vi "Mark as Source Only.vi"() -> ()   [LabVIEW 2011]
uses:
  <vilib>/regexp/Match Regular Expression.xnode
panel:
  in  "Interactive?":bool
  out "errors":path[](array[path])
  out "stripped":path[](array[path])
  out "Progess":i32(slide) scale=0.0..3565.0
  in  "Mark VIs":bool
  in  "IgnoreSVN":bool=TRUE
  in  "Root Folder":path
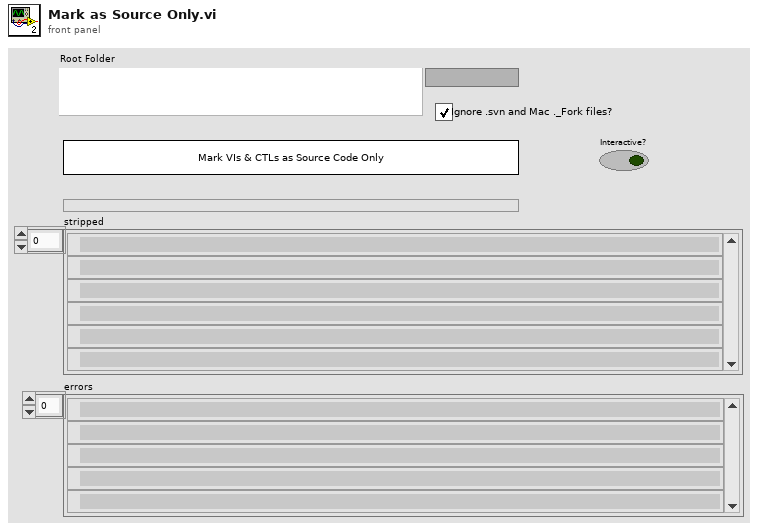
[diagram p1: front panel]
types:
  T1 = enum32{"invalid VI type", "Standard VI", "Control VI", "Global VI", "Polymorphic VI", "Configuration VI", "SubSystem", "Facade VI", "Method VI", "Statechart Diagram VI"}[]
  T2 = enum32{"invalid VI type", "Standard VI", "Control VI", "Global VI", "Polymorphic VI", "Configuration VI", "SubSystem", "Facade VI", "Method VI", "Statechart Diagram VI"}
  T3 = enum16{"Left Button", "Center Button", "Right Button", "Window Close"}
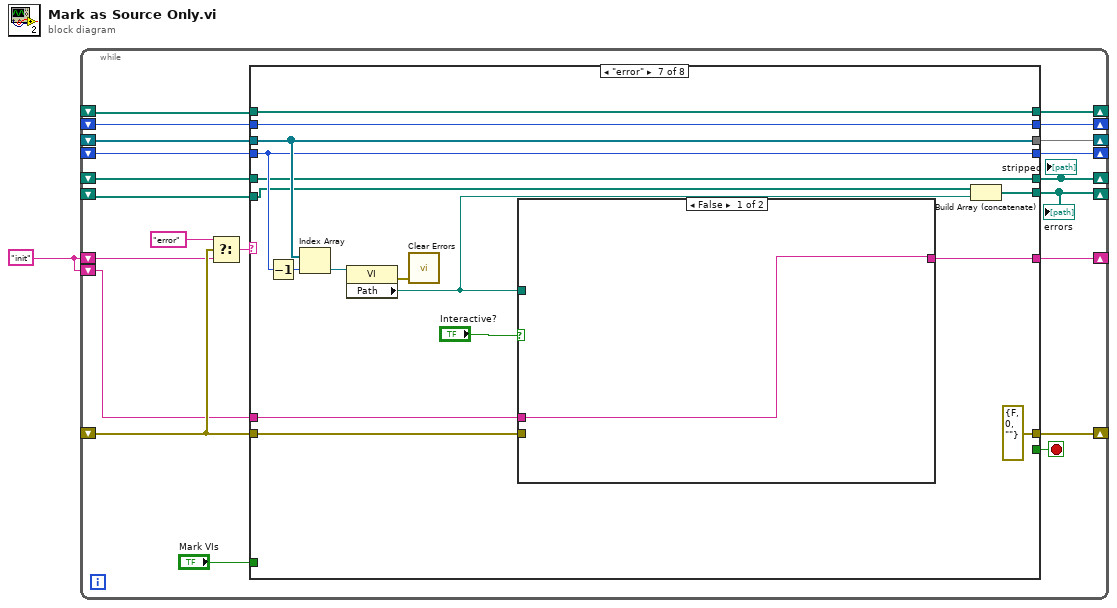
[diagram p0: block diagram]
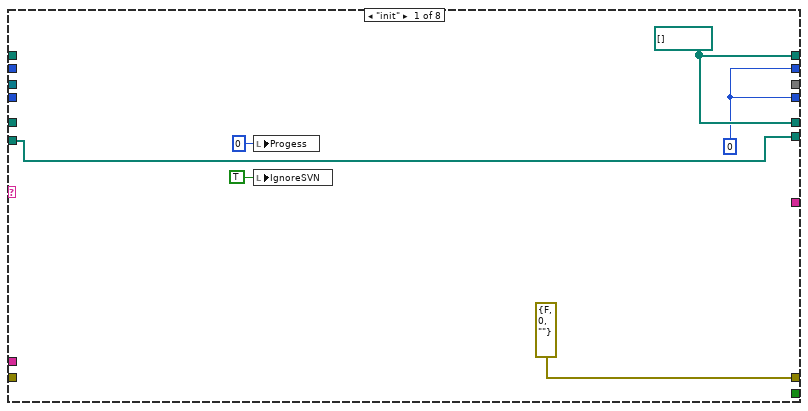
[diagram p2: hidden frame]
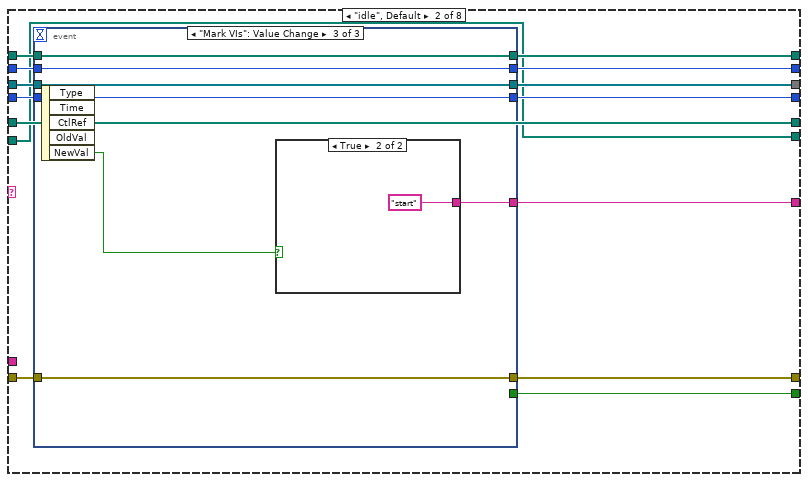
[diagram p3: hidden frame]
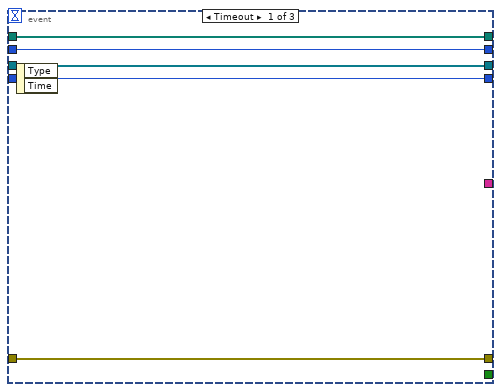
[diagram p4: hidden frame]
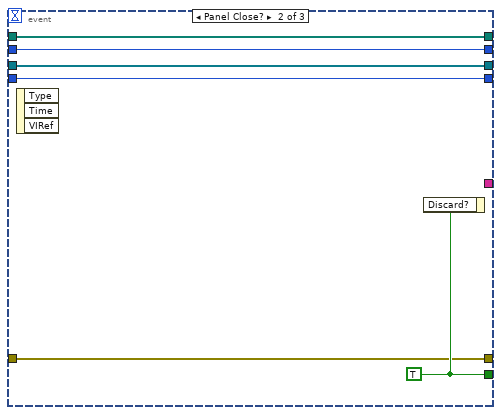
[diagram p5: hidden frame]
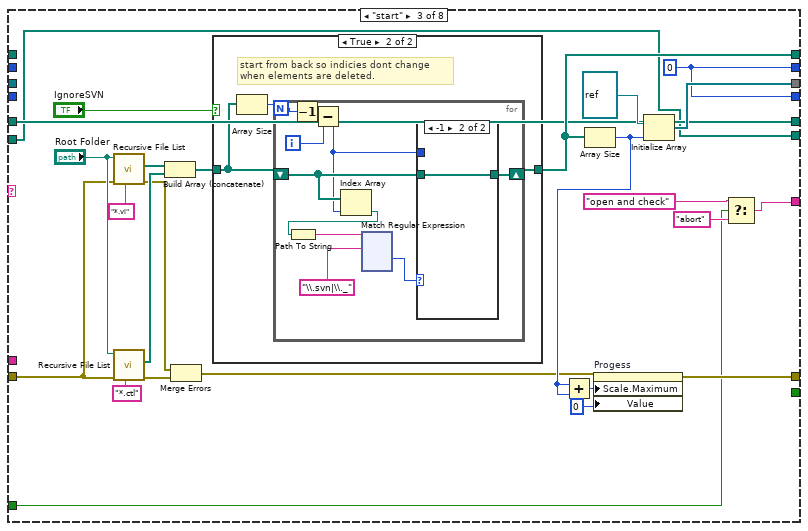
[diagram p7: hidden frame]
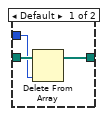
[diagram p9: hidden frame]
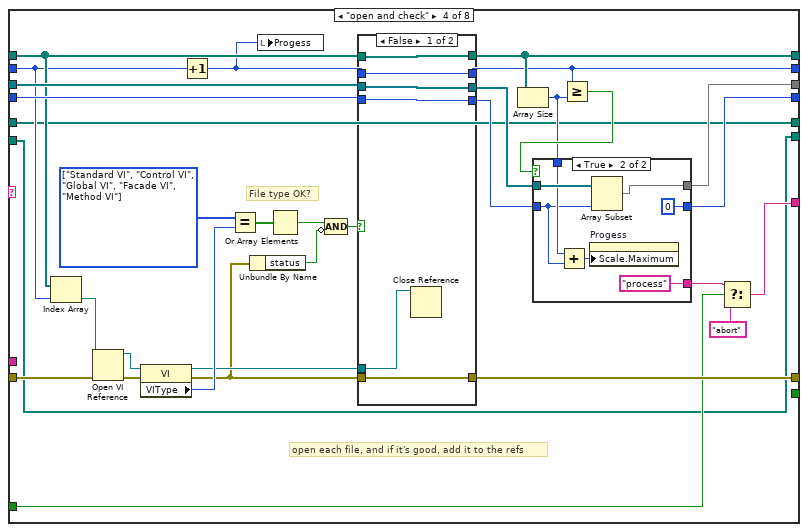
[diagram p10: hidden frame]
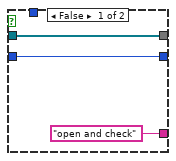
[diagram p11: hidden frame]
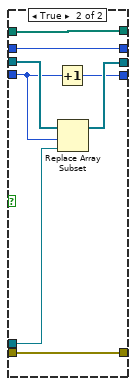
[diagram p12: hidden frame]
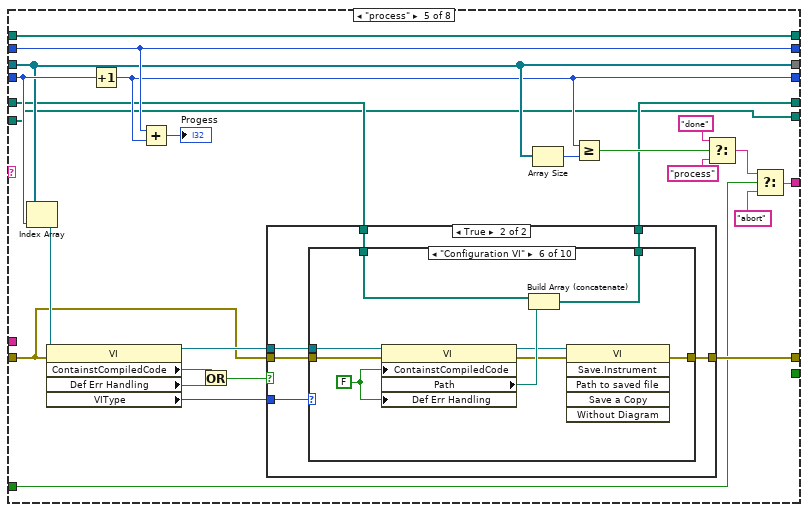
[diagram p13: hidden frame]
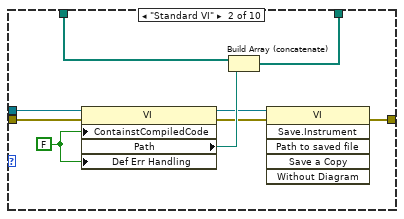
[diagram p16: hidden frame]
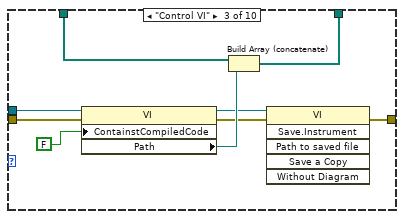
[diagram p17: hidden frame]
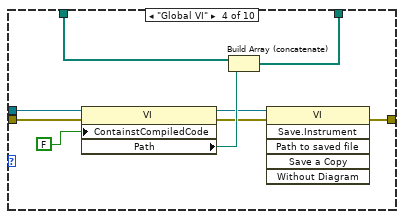
[diagram p18: hidden frame]
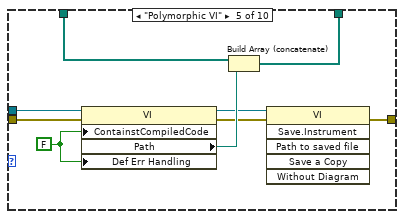
[diagram p19: hidden frame]
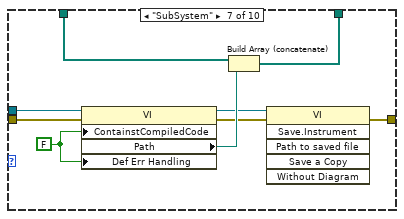
[diagram p20: hidden frame]
diagram:
  w1 = "init"
  n1 = while {
    shift-right: [w17] -> _
    shift-left: w1 -> [w6]
    shift-right: [w18] -> _
    shift-left: _ -> [w19]
    shift-right: [w16] -> _
    shift-left: _ -> [w15]
    shift-right: [w13] -> _
    shift-left: _ -> [w14]
    shift-right: [w12] -> _
    shift-left: _ -> [w11]
    shift-right: [w9] -> _
    shift-left: _ -> [w10]
    shift-left: w1 -> [w7]
    shift-right: [w4] -> _
    shift-left: _ -> [w5]
    shift-right: [w3] -> _
    shift-left: _ -> [w2]
    stop <- w22 stop-if-true
    n2 = Select(t="error", s=w19, f=w6) -> (s? t:f=w20:string)
    n3 = case shown="\"error\"" w20 {
      tunnel: [_ w42 _ _ _ _ _ _] -> w22
      tunnel: w19 -> [_ w41 w72 w247 w273 w395 w406 w432]
      tunnel: [errorcluster {"status"=FALSE, "code"=0, "source"=""} ("error in") w40 w81 w233 w292 w393 errorcluster {"status"=FALSE, "code"=0, "source"=""} ("error out") w430] -> w18
      tunnel: [_ w39 w65 w219 w284 _ w404 _] -> w17
      tunnel: [w26 w36 w68 w230 w293 _ w411 w429] -> w16
      tunnel: w15 -> [_ w38 _ w234 w293 _ w411 w429]
      tunnel: w14 -> [_ w37 _ w231 w294 _ w410 _]
      tunnel: [w25 w35 w75 w226 w294 _ w410 _] -> w13
      tunnel: [_ w34 w78 w224 w291 _ w408 _] -> w12
      tunnel: w11 -> [_ w33 _ w240 w291 w394 w408 w433]
      tunnel: w10 -> [_ w32 _ w238 w296 _ w403 _]
      tunnel: [w25 w31 w75 w227 w289 _ w403 _] -> w9
      tunnel: "Mark VIs" -> [_ _ w64 w221 w282 _ _ _]
      tunnel: w7 -> [_ _ _ _ _ _ w401 _]
      tunnel: w5 -> [_ w30 w63 w217 w279 w389 w400 w428]
      tunnel: [w26 w30 w63 w217 w278 w389 w400 w428] -> w4
      tunnel: [w23 w29 w62 w216 w272 w388 w399 w427] -> w3
      tunnel: w2 -> [w23 w29 w62 w216 w272 w388 w397 w427]
      frame "init" {
        w25 = 0
        w26 = path[] []
        n4 = local write "Progess"(0 ("Progess")) -> ()
        n5 = local write "IgnoreSVN"(TRUE ("IgnoreSVN")) -> ()
      }
      frame "idle", Default {
        n6 = event shown="[2] \"Mark VIs\": Value Change" {
          selector: _ -> [_ _ _]
          dyn-events: _ -> [_ _ _]
          timeout: _ -> [_ _ _]
          tunnel: [_ w53 _] -> w42
          tunnel: w41 -> [w47 w52 w60]
          tunnel: [w47 w52 w60] -> w40
          tunnel: [_ _ w59] -> w39
          tunnel: w38 -> [w45 w51 w57]
          tunnel: w37 -> [w46 w50 w58]
          tunnel: [w45 w51 w57] -> w36
          tunnel: [w46 w50 w58] -> w35
          tunnel: [w43 w49 w55] -> w34
          tunnel: w33 -> [w43 w49 w55]
          tunnel: w32 -> [w44 w48 w56]
          tunnel: [w44 w48 w56] -> w31
          event Timeout {
            n7 = event-data() -> ()  [unwired: 1 in, 2 out]
          }
          event Panel Close? {
            w53 = TRUE
            n8 = event-data() -> ()  [unwired: 1 in, 3 out]
            n9 = event-data("Discard?"=w53) -> ()  [unwired: 1 in, 1 out]
          }
          event "Mark VIs": Value Change {
            n10 = event-data() -> ("NewVal"=w54:bool)  [unwired: 1 in, 4 out]
            n11 = case shown="True" w54 {
              tunnel: [_ "start"] -> w59
              frame False {
              }
              frame True {
              }
            }
          }
        }
      }
      frame "start" {
        w75 = 0
        n12 = call <vilib>:"Recursive File List.vi"("pattern"="*.vi", "error in (no error)"=w72, "Folder Path"="Root Folder") -> ("error out"=w73:errorcluster, "All Files in Dir"=w83:path[])  [unwired: 4 in, 3 out]
        n13 = call <vilib>:"Recursive File List.vi"("pattern"="*.ctl", "error in (no error)"=w72, "Folder Path"="Root Folder") -> ("error out"=w71:errorcluster, "All Files in Dir"=w82:path[])  [unwired: 4 in, 3 out]
        n14 = Build Array (concatenate)(w83, w82) -> (w74:path[])
        n15 = Merge Errors(w73, w71) -> (w70:errorcluster)
        n16 = case shown="True" "IgnoreSVN" {
          tunnel: w74 -> [w87 w88]
          tunnel: [w87 w90] -> w68
          frame False {
          }
          frame True {
            # "start from back so indicies dont change\nwhen elements are deleted."
            n17 = Array Size(array=w88) -> (size(s)=w89:i32)
            n18 = for {
              N: w89 -> [w100]
              shift-right: [w95] -> w90
              shift-left: w88 -> [w97]
              i -> [w99]
              n19 = Decrement(x=w100) -> (x-1=w94:i32)
              n20 = Subtract(x=w94, y=w99) -> (x-y=w96:i32)
              n21 = Index Array(array=w97, index=w96) -> (element=w98:path)
              n22 = Path To String(path=w98) -> (string=w93:string)
              n23 = xnode "Match Regular Expression"("input string"=w93, "regular expression"="\\.svn|\\._") -> ("offset past match"=w92:i32)  [unwired: 4 in, 4 out]
              n24 = case shown="-1" w92 {
                tunnel: w97 -> [w214 w215]
                tunnel: w96 -> [w212 _]
                tunnel: [w213 w215] -> w95
                frame Default {
                  n25 = Delete From Array(array=w214, index=w212) -> (array with subset deleted=w213:path[])  [unwired: 1 in, 1 out]
                }
                frame -1 {
                }
              }
            }
          }
        }
        n26 = Array Size(array=w68) -> (size(s)=w76:i32)
        n27 = Add(x=w76, y=w76) -> (x+y=w77:i32)
        n28 = property on="Progess" class="Slide (strict)"(error in=w70, "Scale.Maximum"=w77, "Value"=0 ("Progess")) -> (error out=w81:errorcluster)  [unwired: 1 in, 1 out]
        n29 = Initialize Array(refnum<vi> refnum ("This VI"), w76) -> (w78:refnum<vi>[])
        n30 = Select(t="open and check", s=w64, f="abort") -> (s? t:f=w65:string)
      }
      frame "open and check" {
        w242 = T1 [enum."Standard VI", enum."Control VI", enum."Global VI", enum."Facade VI", enum."Method VI"] items=["invalid VI type", "Standard VI", "Control VI", "Global VI", "Polymorphic VI", "Configuration VI", "SubSystem", "Facade VI", "Method VI", "Statechart Diagram VI"]
        # "open each file, and if it's good, add it to the refs"
        # "File type OK?"
        n31 = Index Array(array=w234, index=w231) -> (element=w246:path)
        n32 = Open VI Reference(vi path=w246, error in (no error)=w247) -> (vi reference=w244:refnum<vi>, error out=w245:errorcluster)  [unwired: 4 in]
        n33 = property class="VI"(reference=w244, error in=w245) -> (reference out=w239:refnum<vi>, error out=w232:errorcluster, "VIType"=w243:T2)
        n34 = Increment(x=w231) -> (x+1=w225:i32)
        n35 = Equal?(x=w242, y=w243) -> (x = y?=w241:bool[])
        n36 = Unbundle By Name(w232) -> ("status"=w236:bool)
        n37 = local write "Progess"(w225) -> ()
        n38 = Or Array Elements(Boolean array=w241) -> (logical OR=w237:bool)
        n39 = Compound Arithmetic op=AND(w237, invert w236) -> (w235:bool)
        n40 = case shown="False" w235 {
          tunnel: w240 -> [w261 w271]
          tunnel: w239 -> [w259 w270]
          tunnel: [w261 w269] -> w228
          tunnel: w238 -> [w260 w268]
          tunnel: [w260 w267] -> w223
          tunnel: w234 -> [w263 w266]
          tunnel: [w263 w266] -> w230
          tunnel: [w262 w265] -> w226
          tunnel: w225 -> [w262 w265]
          tunnel: [w258 w264] -> w233
          tunnel: w232 -> [w258 w264]
          frame False {
            n41 = Close Reference(reference=w259) -> ()  [unwired: 1 in, 1 out]
          }
          frame True {
            n42 = Increment(x=w268) -> (x+1=w267:i32)
            n43 = Replace Array Subset(array=w271, new element=w270, index=w268) -> (w269:refnum<vi>[])
          }
        }
        n44 = Array Size(array=w230) -> (size(s)=w222:i32)
        n45 = Greater Or Equal?(x=w226, y=w222) -> (x >= y?=w229:bool)
        n46 = case shown="True" w229 {
          tunnel: w228 -> [w250 w255]
          tunnel: w223 -> [w249 w251]
          tunnel: [w250 w254] -> w224
          tunnel: [w249 0] -> w227
          tunnel: ["open and check" "process"] -> w218
          tunnel: w222 -> [_ w252]
          frame False {
          }
          frame True {
            n47 = Add(x=w252, y=w251) -> (x+y=w256:i32)
            n48 = property on="Progess" class="Slide (strict)"("Scale.Maximum"=w256) -> ()  [unwired: 2 in, 2 out]
            n49 = Array Subset(array=w255, length=w251) -> (w254:refnum<vi>[])  [unwired: 1 in]
          }
        }
        n50 = Select(t=w218, s=w221, f="abort") -> (s? t:f=w219:string)
      }
      frame "process" {
        n51 = Index Array(array=w291, index=w296) -> (element=w281:refnum<vi>)
        n52 = property class="VI"(reference=w281, error in=w273) -> (reference out=w280:refnum<vi>, "ContainstCompiledCode"=w276:bool, "Def Err Handling"=w275:bool, "VIType"=w274:T2)  [unwired: 1 out]
        n53 = Increment(x=w296) -> (x+1=w289:i32)
        n54 = Add(x=w294, y=w289) -> (x+y=→"Progess":i32)
        n55 = Or(x=w276, y=w275) -> (x .or. y?=w277:bool)
        n56 = case shown="True" w277 {
          tunnel: [w298 w304] -> w292
          tunnel: w280 -> [_ w303]
          tunnel: w273 -> [w298 w302]
          tunnel: w279 -> [w297 w301]
          tunnel: [w297 w300] -> w278
          tunnel: w274 -> [_ w299]
          frame False {
          }
          frame True {
            n57 = case shown="\"Configuration VI\"" w299 {
              tunnel: [w305 w315 w324 w333 w342 w351 w360 w369 w378 w387] -> w304
              tunnel: w303 -> [_ w314 w323 w332 w341 w350 w359 w368 w377 w386]
              tunnel: w302 -> [w305 w313 w322 w331 w340 w349 w358 w367 w376 w385]
              tunnel: w301 -> [w306 w312 w321 w330 w339 w348 w357 w366 w375 w384]
              tunnel: [w306 w310 w319 w328 w337 w346 w355 w364 w373 w382] -> w300
              frame "invalid VI type", Default {
              }
              frame "Standard VI" {
                w307 = FALSE ("Contains Compiled Code")
                n58 = property class="VI"(reference=w314, error in=w313, "ContainstCompiledCode"=w307, "Def Err Handling"=w307) -> (reference out=w309:refnum<vi>, error out=w308:errorcluster, "Path"=w311:path)
                n59 = Build Array (concatenate)(w312, w311) -> (w310:path[])
                n60 = invoke class="VI" method="Save.Instrument"(reference=w309, error in=w308) -> (error out=w315:errorcluster)  [unwired: 4 in, 5 out]
              }
              frame "Control VI" {
                n61 = property class="VI"(reference=w323, error in=w322, "ContainstCompiledCode"=FALSE ("Contains Compiled Code")) -> (reference out=w318:refnum<vi>, error out=w317:errorcluster, "Path"=w320:path)
                n62 = Build Array (concatenate)(w321, w320) -> (w319:path[])
                n63 = invoke class="VI" method="Save.Instrument"(reference=w318, error in=w317) -> (error out=w324:errorcluster)  [unwired: 4 in, 5 out]
              }
              frame "Global VI" {
                n64 = property class="VI"(reference=w332, error in=w331, "ContainstCompiledCode"=FALSE ("Contains Compiled Code")) -> (reference out=w327:refnum<vi>, error out=w326:errorcluster, "Path"=w329:path)
                n65 = Build Array (concatenate)(w330, w329) -> (w328:path[])
                n66 = invoke class="VI" method="Save.Instrument"(reference=w327, error in=w326) -> (error out=w333:errorcluster)  [unwired: 4 in, 5 out]
              }
              frame "Polymorphic VI" {
                w334 = FALSE ("Contains Compiled Code")
                n67 = property class="VI"(reference=w341, error in=w340, "ContainstCompiledCode"=w334, "Def Err Handling"=w334) -> (reference out=w336:refnum<vi>, error out=w335:errorcluster, "Path"=w338:path)
                n68 = Build Array (concatenate)(w339, w338) -> (w337:path[])
                n69 = invoke class="VI" method="Save.Instrument"(reference=w336, error in=w335) -> (error out=w342:errorcluster)  [unwired: 4 in, 5 out]
              }
              frame "Configuration VI" {
                w343 = FALSE ("Contains Compiled Code")
                n70 = property class="VI"(reference=w350, error in=w349, "ContainstCompiledCode"=w343, "Def Err Handling"=w343) -> (reference out=w345:refnum<vi>, error out=w344:errorcluster, "Path"=w347:path)
                n71 = Build Array (concatenate)(w348, w347) -> (w346:path[])
                n72 = invoke class="VI" method="Save.Instrument"(reference=w345, error in=w344) -> (error out=w351:errorcluster)  [unwired: 4 in, 5 out]
              }
              frame "SubSystem" {
                w352 = FALSE ("Contains Compiled Code")
                n73 = property class="VI"(reference=w359, error in=w358, "ContainstCompiledCode"=w352, "Def Err Handling"=w352) -> (reference out=w354:refnum<vi>, error out=w353:errorcluster, "Path"=w356:path)
                n74 = Build Array (concatenate)(w357, w356) -> (w355:path[])
                n75 = invoke class="VI" method="Save.Instrument"(reference=w354, error in=w353) -> (error out=w360:errorcluster)  [unwired: 4 in, 5 out]
              }
              frame "Facade VI" {
                w361 = FALSE ("Contains Compiled Code")
                n76 = property class="VI"(reference=w368, error in=w367, "ContainstCompiledCode"=w361, "Def Err Handling"=w361) -> (reference out=w363:refnum<vi>, error out=w362:errorcluster, "Path"=w365:path)
                n77 = Build Array (concatenate)(w366, w365) -> (w364:path[])
                n78 = invoke class="VI" method="Save.Instrument"(reference=w363, error in=w362) -> (error out=w369:errorcluster)  [unwired: 4 in, 5 out]
              }
              frame "Method VI" {
                w370 = FALSE ("Contains Compiled Code")
                n79 = property class="VI"(reference=w377, error in=w376, "ContainstCompiledCode"=w370, "Def Err Handling"=w370) -> (reference out=w372:refnum<vi>, error out=w371:errorcluster, "Path"=w374:path)
                n80 = Build Array (concatenate)(w375, w374) -> (w373:path[])
                n81 = invoke class="VI" method="Save.Instrument"(reference=w372, error in=w371) -> (error out=w378:errorcluster)  [unwired: 4 in, 5 out]
              }
              frame "Statechart Diagram VI" {
                w379 = FALSE ("Contains Compiled Code")
                n82 = property class="VI"(reference=w386, error in=w385, "ContainstCompiledCode"=w379, "Def Err Handling"=w379) -> (reference out=w381:refnum<vi>, error out=w380:errorcluster, "Path"=w383:path)
                n83 = Build Array (concatenate)(w384, w383) -> (w382:path[])
                n84 = invoke class="VI" method="Save.Instrument"(reference=w381, error in=w380) -> (error out=w387:errorcluster)  [unwired: 4 in, 5 out]
              }
            }
          }
        }
        n85 = Array Size(array=w291) -> (size(s)=w290:i32)
        n86 = Greater Or Equal?(x=w289, y=w290) -> (x >= y?=w288:bool)
        n87 = Select(t="done", s=w288, f="process") -> (s? t:f=w285:string)
        n88 = Select(t=w285, s=w282, f="abort") -> (s? t:f=w284:string)
      }
      frame "done" {
        n89 = Close Reference(reference=w394, error in (no error)=w395) -> (error out=w393:errorcluster)
        n90 = property on="Progess" class="Slide (strict)"() -> ("Scale.Maximum"=w392:dbl)  [unwired: 2 in, 2 out]
        n91 = local write "Progess"(w392) -> ()
        n92 = local write "Mark VIs"(FALSE ("Mark VIs")) -> ()
        n93 = One Button Dialog(message="Finished!") -> ()  [unwired: 1 in, 1 out]
      }
      frame "error" {
        n94 = Decrement(x=w403) -> (x-1=w407:i32)
        n95 = Index Array(array=w408, index=w407) -> (element=w409:refnum<vi>)
        n96 = property class="VI"(reference=w409) -> (error out=w405:errorcluster, "Path"=w398:path)  [unwired: 1 in, 1 out]
        n97 = call <vilib>:"Clear Errors.vi"("error in (no error)"=w405) -> ()  [unwired: 6 in, 1 out]
        n98 = case shown="False" "Interactive?" {
          tunnel: w406 -> [_ w419]
          tunnel: [w412 w415] -> w404
          tunnel: w401 -> [w412 w414]
          tunnel: w398 -> [_ w413]
          frame False {
          }
          frame True {
            n99 = Format Into String(format string="\"%s\"\nCould not be marked as Source Code Only!\n\nView error message?", w413) -> (resulting string=w421:string)  [unwired: 2 in, 1 out]
            n100 = call <vilib>:"Three Button Dialog.vi"("Right Button Text (\"Cancel\")"="Abort" ("Right Button Text (\"Cancel\")"), "Center Button Text (\"No\")"="No" ("F button name (\"Cancel\")"), "Left Button Text (\"Yes\")"="Yes" ("T button name (\"OK\")"), "message"=w421) -> ("Which Button?"=w420:T3)  [unwired: 7 in]
            n101 = case shown="\"Left Button\"" w420 {
              tunnel: w419 -> [w424 _ _]
              tunnel: [w423 w425 "abort"] -> w415
              tunnel: w414 -> [w423 w425 _]
              frame "Left Button" {
                n102 = call <vilib>:"Simple Error Handler.vi"("error source (\" \")"=w423, "error in (no error)"=w424) -> ()  [unwired: 3 in, 5 out]
              }
              frame "Center Button", Default {
              }
              frame "Right Button" {
              }
            }
          }
        }
        n103 = Build Array (concatenate)(w397, w398) -> (w399:path[])
      }
      frame "abort" {
        n104 = Close Reference(reference=w433, error in (no error)=w432) -> (error out=w431:errorcluster)
        n105 = call <vilib>:"Clear Errors.vi"("error in (no error)"=w431) -> ("error out"=w430:errorcluster)  [unwired: 6 in]
        n106 = One Button Dialog(message="operation aborted.") -> ()  [unwired: 1 in, 1 out]
        n107 = local write "Mark VIs"(FALSE ("Mark VIs")) -> ()
      }
    }
    "stripped" <- w4
    "errors" <- w3
  }
